vi "temperature.vi"(3 "Stop Button":bool, 4 "Temp2 Port":tag="Dev2", 5 "Temp1 Port":tag="Dev1") -> (0 "Delta T":dbl, 1 "Temp2":dbl, 2 "Temp1":dbl)   [LabVIEW 2013]
panel:
  out "Temperature":cluster{"Scalar":dbl, "Scalar":dbl, dbl}(graph)
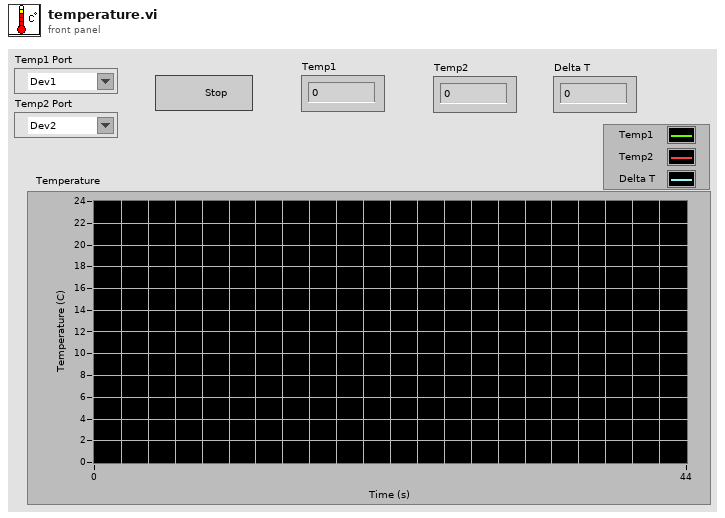
[diagram p1: front panel]
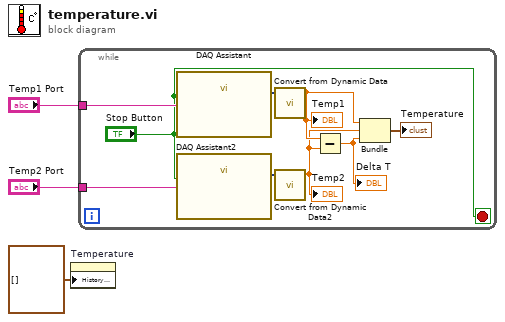
[diagram p0: block diagram]
diagram:
  n1 = property on="Temperature" class="WFChart (strict)"("History Data"=cluster{"Scalar":dbl, "Scalar":dbl, dbl}[] []) -> ()  [unwired: 2 in, 2 out]
  n2 = while {
    tunnel: "Temp1 Port" -> [w12]
    tunnel: "Temp2 Port" -> [w11]
    stop <- "Stop Button" stop-if-true
    n3 = call "DAQ Assistant"("stop (T)"="Stop Button", "device name"=w12) -> ("data"=w8:dynamicdata)  [unwired: 15 in, 2 out]
    n4 = call "DAQ Assistant2"("stop (T)"="Stop Button", "device name"=w11) -> ("data"=w9:dynamicdata)  [unwired: 15 in, 2 out]
    n5 = call "Convert from Dynamic Data"("Dynamic Data Type"=w8) -> ("Scalar"=w7:dbl)  [unwired: 3 in]
    "Temp1" <- w7
    n6 = call "Convert from Dynamic Data2"("Dynamic Data Type"=w9) -> ("Scalar"=w6:dbl)  [unwired: 3 in]
    "Temp2" <- w6
    n7 = Subtract(x=w7, y=w6) -> (x-y=w5:dbl)
    "Delta T" <- w5
    n8 = Bundle("Scalar"=w7, "Scalar"=w6, w5) -> (→"Temperature":cluster{"Scalar":dbl, "Scalar":dbl, dbl})  [unwired: 1 in]
  }
